vi "ControlKeithley2614.vi"() -> ()   [LabVIEW 2017]
panel:
  in  "GPIB Address":string="12"
  out "String":string
  in  "Record new values":bool
  out "Output Current (A)":dbl
  out "Output Voltage (V)":dbl
  out "Compliance limit (V)":dbl
  out "Current Range":u16(ring) items=["100 nA", "1 uA", "10 uA", "100 uA", "1 mA", "10 mA", "100 mA", "1 A"]
  out "Voltage Range":u16(ring) items=["200 mV", "2 V", "20 V", "200 V"]
  out "Current (sourse)":dbl
  out "Voltage (sourse)":dbl
  out "ComplianceIndicator":bool
  out "Compliance limit (A)":dbl
  out "Source Function":u16(ring)=1 items=["Current Source", "Voltage Source"]
  out "Sence Mode":u16(ring) items=["2-wire", "4-wire"]
  in  "ON/OFF channel":bool
  out "ON/OFF indicator":bool
  in  "error in (no error)":errorcluster
  out "error out":errorcluster
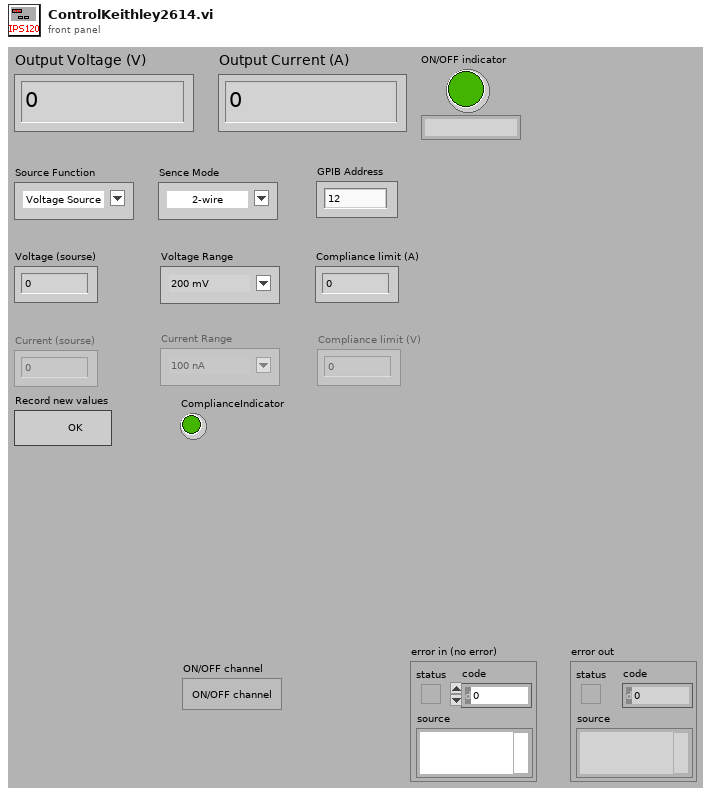
[diagram p1: front panel]
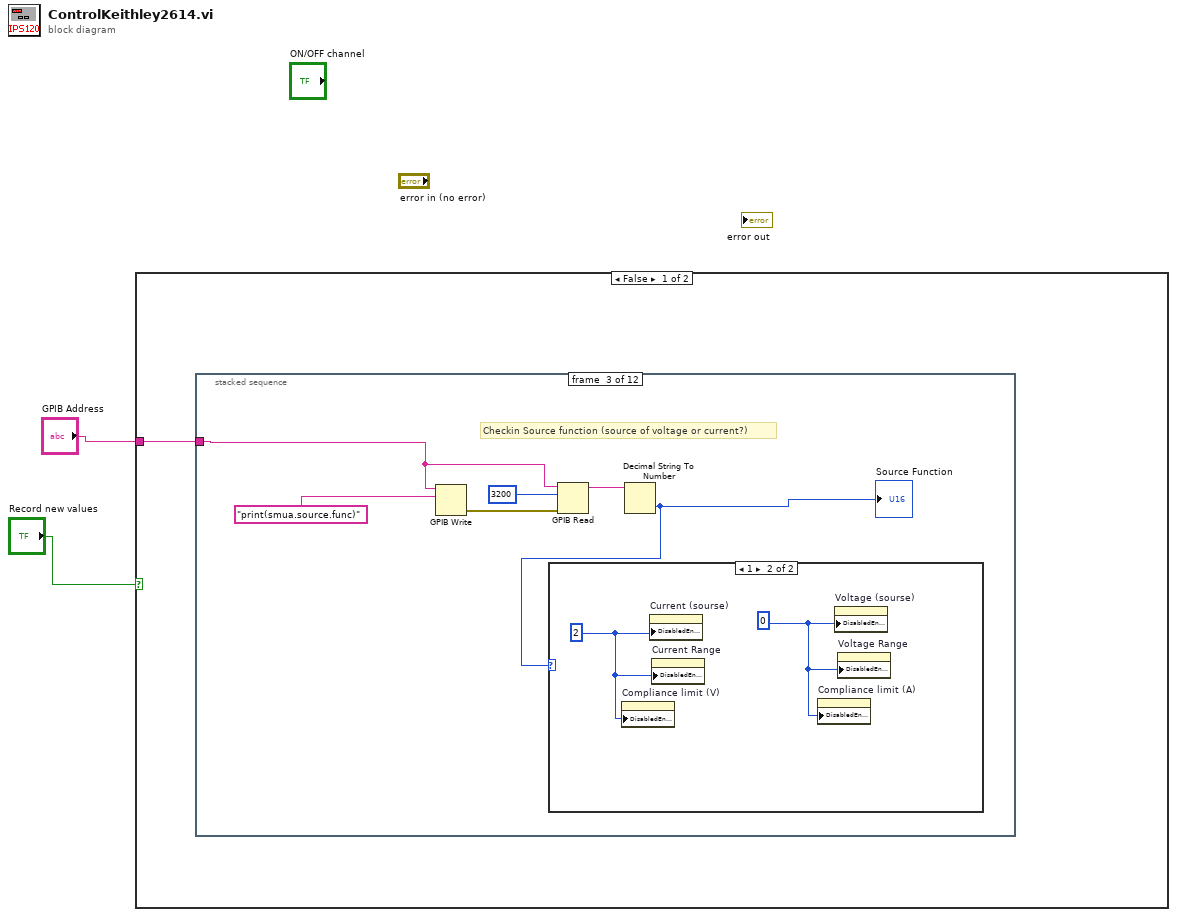
[diagram p0: block diagram]
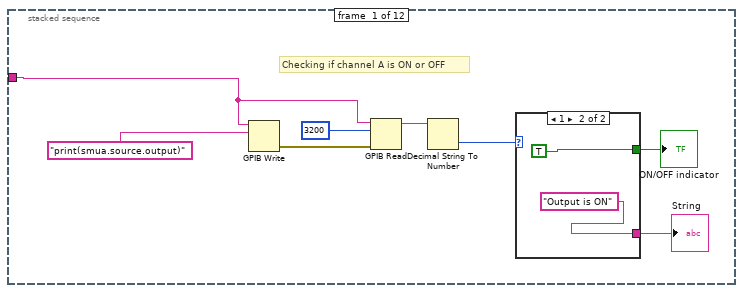
[diagram p2: hidden frame]
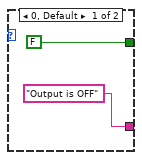
[diagram p3: hidden frame]
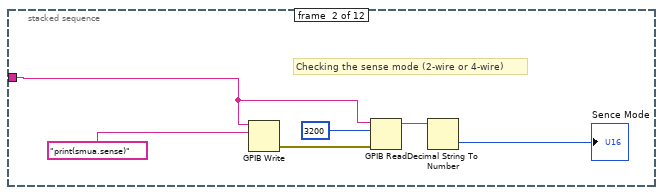
[diagram p4: hidden frame]
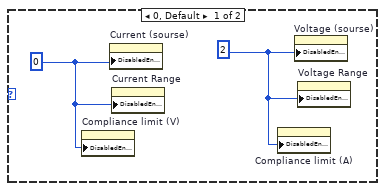
[diagram p5: hidden frame]
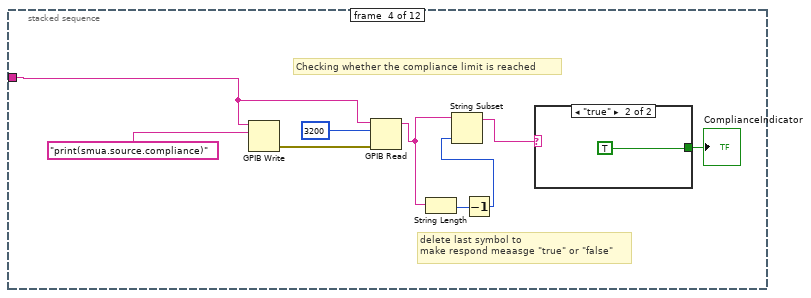
[diagram p6: hidden frame]
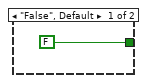
[diagram p7: hidden frame]
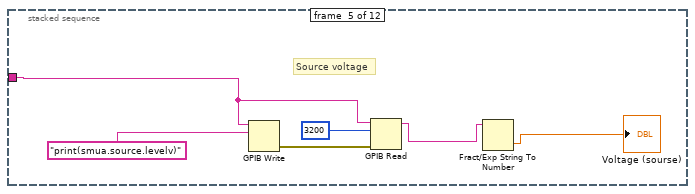
[diagram p8: hidden frame]
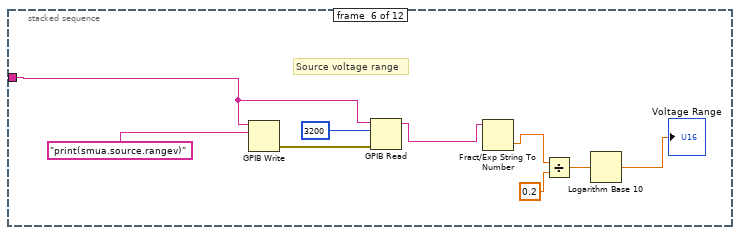
[diagram p9: hidden frame]
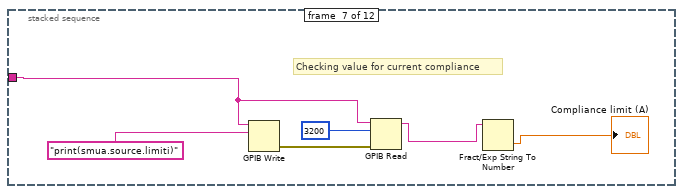
[diagram p10: hidden frame]
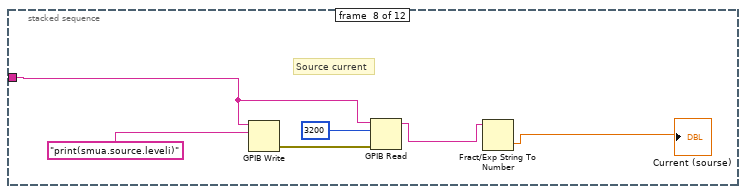
[diagram p11: hidden frame]
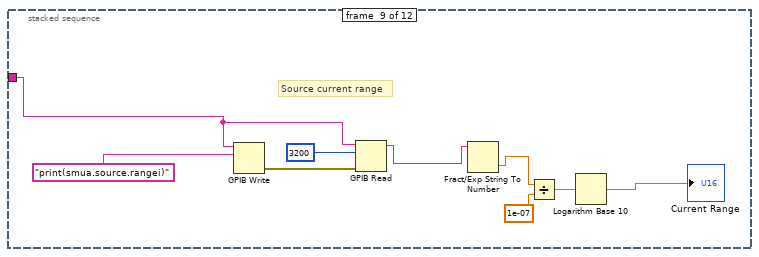
[diagram p12: hidden frame]
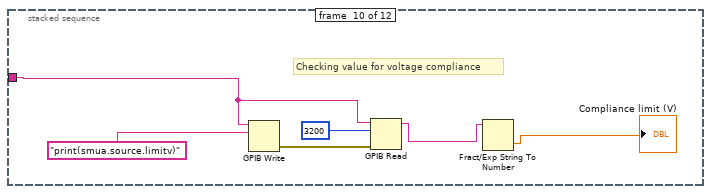
[diagram p13: hidden frame]
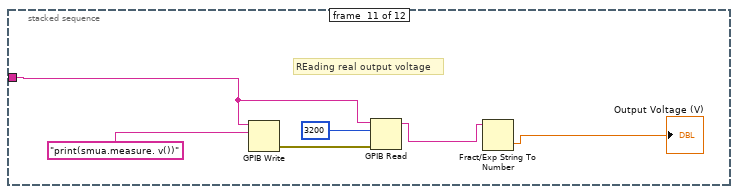
[diagram p14: hidden frame]
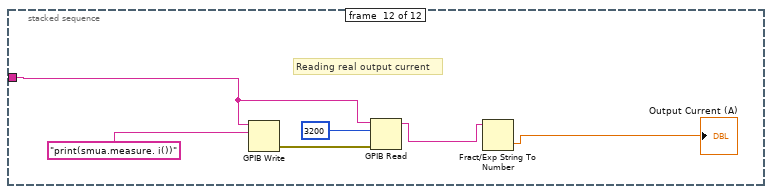
[diagram p15: hidden frame]
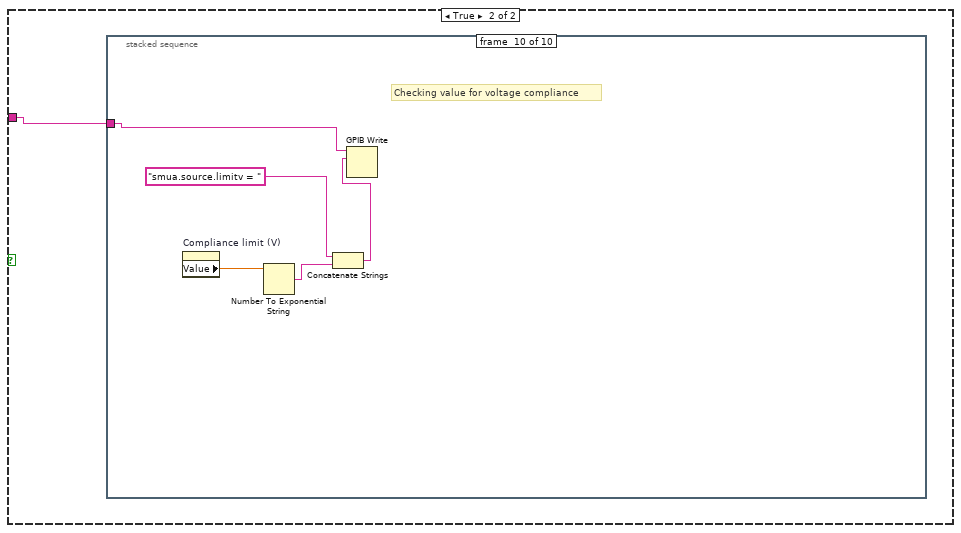
[diagram p16: hidden frame]
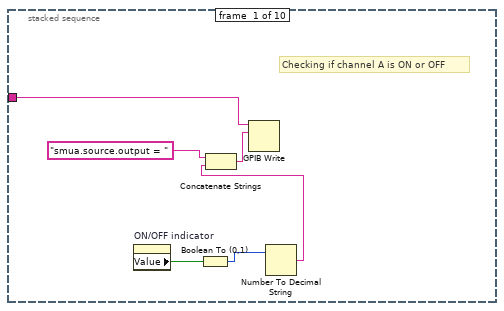
[diagram p17: hidden frame]
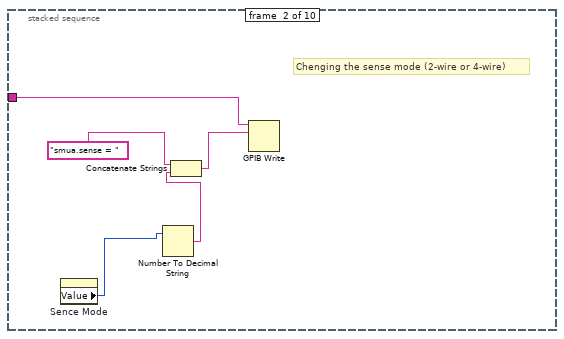
[diagram p18: hidden frame]
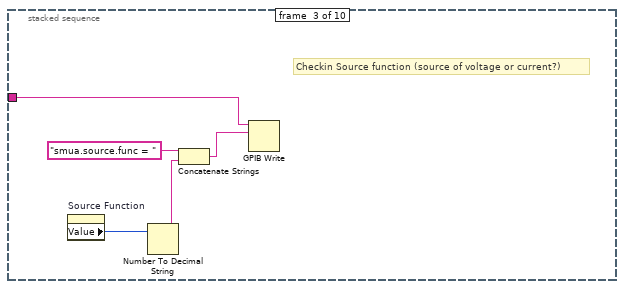
[diagram p19: hidden frame]
diagram:
  n1 = case shown="False" "Record new values" {
    tunnel: "GPIB Address" -> [w3 w97]
    frame False {
      n2 = stacked-sequence {
        tunnel: w3 -> [w4 w16 w22 w32 w43 w49 w58 w64 w70 w79 w85 w91]
        frame #0 {
          # "Checking if channel A is ON or OFF"
          n3 = GPIB Write(0:w4, 1:"print(smua.source.output)") -> (6:w11:errorcluster)  [unwired: 3 in, 1 out]
          n4 = GPIB Read(0:w4, 1:3200, 3:w11) -> (5:w8:string)  [unwired: 2 in, 2 out]
          n5 = Decimal String To Number(string=w8) -> (number=w7:i32)  [unwired: 2 in, 1 out]
          n6 = case shown="1" w7 {
            tunnel: [FALSE TRUE] -> w6
            tunnel: ["Output is OFF" "Output is ON"] -> w5
            frame 0, Default {
            }
            frame 1 {
            }
          }
          "ON/OFF indicator" <- w6
          "String" <- w5
        }
        frame #1 {
          # "Checking the sense mode (2-wire or 4-wire)"
          n7 = GPIB Write(0:w16, 1:"print(smua.sense)") -> (6:w21:errorcluster)  [unwired: 3 in, 1 out]
          n8 = GPIB Read(0:w16, 1:3200, 3:w21) -> (5:w18:string)  [unwired: 2 in, 2 out]
          n9 = Decimal String To Number(string=w18) -> (number=→"Sence Mode":i32)  [unwired: 2 in, 1 out]
        }
        frame #2 {
          # "Checkin Source function (source of voltage or current?)"
          n10 = GPIB Write(0:w22, 1:"print(smua.source.func)") -> (6:w27:errorcluster)  [unwired: 3 in, 1 out]
          n11 = GPIB Read(0:w22, 1:3200, 3:w27) -> (5:w24:string)  [unwired: 2 in, 2 out]
          n12 = Decimal String To Number(string=w24) -> (number=w23:i32)  [unwired: 2 in, 1 out]
          "Source Function" <- w23
          n13 = case shown="1" w23 {
            frame 0, Default {
              w28 = 2
              w29 = 0
              n14 = property on="Compliance limit (V)" class="DigNum (strict)"("DisabledEnum"=w29) -> ()  [unwired: 2 in, 2 out]
              n15 = property on="Current (sourse)" class="DigNum (strict)"("DisabledEnum"=w29) -> ()  [unwired: 2 in, 2 out]
              n16 = property on="Current Range" class="Ring (strict)"("DisabledEnum"=w29) -> ()  [unwired: 2 in, 2 out]
              n17 = property on="Compliance limit (A)" class="DigNum (strict)"("DisabledEnum"=w28) -> ()  [unwired: 2 in, 2 out]
              n18 = property on="Voltage (sourse)" class="DigNum (strict)"("DisabledEnum"=w28) -> ()  [unwired: 2 in, 2 out]
              n19 = property on="Voltage Range" class="Ring (strict)"("DisabledEnum"=w28) -> ()  [unwired: 2 in, 2 out]
            }
            frame 1 {
              w30 = 0
              w31 = 2
              n20 = property on="Compliance limit (V)" class="DigNum (strict)"("DisabledEnum"=w31) -> ()  [unwired: 2 in, 2 out]
              n21 = property on="Current (sourse)" class="DigNum (strict)"("DisabledEnum"=w31) -> ()  [unwired: 2 in, 2 out]
              n22 = property on="Current Range" class="Ring (strict)"("DisabledEnum"=w31) -> ()  [unwired: 2 in, 2 out]
              n23 = property on="Compliance limit (A)" class="DigNum (strict)"("DisabledEnum"=w30) -> ()  [unwired: 2 in, 2 out]
              n24 = property on="Voltage (sourse)" class="DigNum (strict)"("DisabledEnum"=w30) -> ()  [unwired: 2 in, 2 out]
              n25 = property on="Voltage Range" class="Ring (strict)"("DisabledEnum"=w30) -> ()  [unwired: 2 in, 2 out]
            }
          }
        }
        frame #3 {
          # "delete last symbol to\nmake respond meaasge \"true\" or \"false\""
          # "Checking whether the compliance limit is reached"
          n26 = GPIB Write(0:w32, 1:"print(smua.source.compliance)") -> (6:w40:errorcluster)  [unwired: 3 in, 1 out]
          n27 = GPIB Read(0:w32, 1:3200, 3:w40) -> (5:w34:string)  [unwired: 2 in, 2 out]
          n28 = String Length(string=w34) -> (length=w36:i32)
          n29 = Decrement(x=w36) -> (x-1=w35:i32)
          n30 = String Subset(string=w34, length (rest)=w35) -> (substring=w33:string)  [unwired: 1 in]
          n31 = case shown="\"true\"" w33 {
            tunnel: [FALSE TRUE] -> w37
            frame "False", Default {
            }
            frame "true" {
            }
          }
          "ComplianceIndicator" <- w37
        }
        frame #4 {
          # "Source voltage"
          n32 = GPIB Write(0:w43, 1:"print(smua.source.levelv)") -> (6:w48:errorcluster)  [unwired: 3 in, 1 out]
          n33 = GPIB Read(0:w43, 1:3200, 3:w48) -> (5:w45:string)  [unwired: 2 in, 2 out]
          n34 = Fract/Exp String To Number(string=w45) -> (number=→"Voltage (sourse)":dbl)  [unwired: 3 in, 1 out]
        }
        frame #5 {
          # "Source voltage range"
          n35 = GPIB Write(0:w49, 1:"print(smua.source.rangev)") -> (6:w57:errorcluster)  [unwired: 3 in, 1 out]
          n36 = GPIB Read(0:w49, 1:3200, 3:w57) -> (5:w54:string)  [unwired: 2 in, 2 out]
          n37 = Fract/Exp String To Number(string=w54) -> (number=w52:dbl)  [unwired: 3 in, 1 out]
          n38 = Divide(x=w52, y=0.2) -> (x/y=w51:dbl)
          n39 = Logarithm Base 10(1:w51) -> (0:→"Voltage Range":dbl)
        }
        frame #6 {
          # "Checking value for current compliance"
          n40 = GPIB Write(0:w58, 1:"print(smua.source.limiti)") -> (6:w63:errorcluster)  [unwired: 3 in, 1 out]
          n41 = GPIB Read(0:w58, 1:3200, 3:w63) -> (5:w60:string)  [unwired: 2 in, 2 out]
          n42 = Fract/Exp String To Number(string=w60) -> (number=→"Compliance limit (A)":dbl)  [unwired: 3 in, 1 out]
        }
        frame #7 {
          # "Source current"
          n43 = GPIB Write(0:w64, 1:"print(smua.source.leveli)") -> (6:w69:errorcluster)  [unwired: 3 in, 1 out]
          n44 = GPIB Read(0:w64, 1:3200, 3:w69) -> (5:w66:string)  [unwired: 2 in, 2 out]
          n45 = Fract/Exp String To Number(string=w66) -> (number=→"Current (sourse)":dbl)  [unwired: 3 in, 1 out]
        }
        frame #8 {
          # "Source current range"
          n46 = GPIB Write(0:w70, 1:"print(smua.source.rangei)") -> (6:w78:errorcluster)  [unwired: 3 in, 1 out]
          n47 = GPIB Read(0:w70, 1:3200, 3:w78) -> (5:w75:string)  [unwired: 2 in, 2 out]
          n48 = Fract/Exp String To Number(string=w75) -> (number=w73:dbl)  [unwired: 3 in, 1 out]
          n49 = Divide(x=w73, y=1e-07) -> (x/y=w72:dbl)
          n50 = Logarithm Base 10(1:w72) -> (0:→"Current Range":dbl)
        }
        frame #9 {
          # "Checking value for voltage compliance"
          n51 = GPIB Write(0:w79, 1:"print(smua.source.limitv)") -> (6:w84:errorcluster)  [unwired: 3 in, 1 out]
          n52 = GPIB Read(0:w79, 1:3200, 3:w84) -> (5:w81:string)  [unwired: 2 in, 2 out]
          n53 = Fract/Exp String To Number(string=w81) -> (number=→"Compliance limit (V)":dbl)  [unwired: 3 in, 1 out]
        }
        frame #10 {
          # "REading real output voltage"
          n54 = GPIB Write(0:w85, 1:"print(smua.measure. v())") -> (6:w90:errorcluster)  [unwired: 3 in, 1 out]
          n55 = GPIB Read(0:w85, 1:3200, 3:w90) -> (5:w87:string)  [unwired: 2 in, 2 out]
          n56 = Fract/Exp String To Number(string=w87) -> (number=→"Output Voltage (V)":dbl)  [unwired: 3 in, 1 out]
        }
        frame #11 {
          # "Reading real output current"
          n57 = GPIB Write(0:w91, 1:"print(smua.measure. i())") -> (6:w96:errorcluster)  [unwired: 3 in, 1 out]
          n58 = GPIB Read(0:w91, 1:3200, 3:w96) -> (5:w93:string)  [unwired: 2 in, 2 out]
          n59 = Fract/Exp String To Number(string=w93) -> (number=→"Output Current (A)":dbl)  [unwired: 3 in, 1 out]
        }
      }
    }
    frame True {
      n60 = stacked-sequence {
        tunnel: w97 -> [w98 w104 w109 _ w114 w119 w127 w132 w137 w145]
        frame #0 {
          # "Checking if channel A is ON or OFF"
          n61 = property on="ON/OFF indicator" class="Bool (strict)"() -> ("Value"=w103:bool)  [unwired: 2 in, 2 out]
          n62 = Boolean To (0,1)(Boolean=w103) -> (0, 1=w102:i16)
          n63 = Number To Decimal String(number=w102) -> (decimal integer string=w100:string)  [unwired: 1 in]
          n64 = Concatenate Strings("smua.source.output = ", w100) -> (w99:string)
          n65 = GPIB Write(0:w98, 1:w99) -> ()  [unwired: 3 in, 2 out]
        }
        frame #1 {
          # "Chenging the sense mode (2-wire or 4-wire)"
          n66 = property on="Sence Mode" class="Ring (strict)"() -> ("Value"=w105:u16)  [unwired: 2 in, 2 out]
          n67 = Number To Decimal String(number=w105) -> (decimal integer string=w107:string)  [unwired: 1 in]
          n68 = Concatenate Strings("smua.sense = ", w107) -> (w106:string)
          n69 = GPIB Write(0:w104, 1:w106) -> ()  [unwired: 3 in, 2 out]
        }
        frame #2 {
          # "Checkin Source function (source of voltage or current?)"
          n70 = property on="Source Function" class="Ring (strict)"() -> ("Value"=w112:u16)  [unwired: 2 in, 2 out]
          n71 = Number To Decimal String(number=w112) -> (decimal integer string=w111:string)  [unwired: 1 in]
          n72 = Concatenate Strings("smua.source.func = ", w111) -> (w110:string)
          n73 = GPIB Write(0:w109, 1:w110) -> ()  [unwired: 3 in, 2 out]
        }
        frame #3 {
        }
        frame #4 {
          # "Source voltage"
          n74 = property on="Voltage (sourse)" class="DigNum (strict)"() -> ("Value"=w117:dbl)  [unwired: 2 in, 2 out]
          n75 = Number To Exponential String(number=w117) -> (E-format string=w116:string)  [unwired: 3 in]
          n76 = Concatenate Strings("smua.source.levelv = ", w116) -> (w115:string)
          n77 = GPIB Write(0:w114, 1:w115) -> ()  [unwired: 3 in, 2 out]
        }
        frame #5 {
          # "Source voltage range"
          n78 = property on="Voltage Range" class="Ring (strict)"() -> ("Value"=w126:u16)  [unwired: 2 in, 2 out]
          n79 = Power Of 10(x=w126) -> (10^x=w121:dbl)
          n80 = Multiply(x=w121, y=0.2) -> (x*y=w120:dbl)
          n81 = Number To Exponential String(number=w120) -> (E-format string=w125:string)  [unwired: 3 in]
          n82 = Concatenate Strings("smua.source.rangev = ", w125) -> (w123:string)
          n83 = GPIB Write(0:w119, 1:w123) -> ()  [unwired: 3 in, 2 out]
        }
        frame #6 {
          # "Checking value for current compliance"
          n84 = property on="Compliance limit (A)" class="DigNum (strict)"() -> ("Value"=w131:dbl)  [unwired: 2 in, 2 out]
          n85 = Number To Exponential String(number=w131) -> (E-format string=w130:string)  [unwired: 3 in]
          n86 = Concatenate Strings("smua.source.limiti = ", w130) -> (w128:string)
          n87 = GPIB Write(0:w127, 1:w128) -> ()  [unwired: 3 in, 2 out]
        }
        frame #7 {
          # "Source current"
          n88 = property on="Current (sourse)" class="DigNum (strict)"() -> ("Value"=w135:dbl)  [unwired: 2 in, 2 out]
          n89 = Number To Exponential String(number=w135) -> (E-format string=w136:string)  [unwired: 3 in]
          n90 = Concatenate Strings("smua.source.leveli = ", w136) -> (w133:string)
          n91 = GPIB Write(0:w132, 1:w133) -> ()  [unwired: 3 in, 2 out]
        }
        frame #8 {
          # "Source current range"
          n92 = property on="Current Range" class="Ring (strict)"() -> ("Value"=w144:u16)  [unwired: 2 in, 2 out]
          n93 = Power Of 10(x=w144) -> (10^x=w143:dbl)
          n94 = Multiply(x=w143, y=1e-07) -> (x*y=w141:dbl)
          n95 = Number To Exponential String(number=w141) -> (E-format string=w140:string)  [unwired: 3 in]
          n96 = Concatenate Strings("smua.source.rangei = ", w140) -> (w138:string)
          n97 = GPIB Write(0:w137, 1:w138) -> ()  [unwired: 3 in, 2 out]
        }
        frame #9 {
          # "Checking value for voltage compliance"
          n98 = property on="Compliance limit (V)" class="DigNum (strict)"() -> ("Value"=w147:dbl)  [unwired: 2 in, 2 out]
          n99 = Number To Exponential String(number=w147) -> (E-format string=w146:string)  [unwired: 3 in]
          n100 = Concatenate Strings("smua.source.limitv = ", w146) -> (w148:string)
          n101 = GPIB Write(0:w145, 1:w148) -> ()  [unwired: 3 in, 2 out]
        }
      }
    }
  }
